vi "LibCam_Open.vi"(7 "webcamnum":i32, 8 "error in (no error)":errorcluster, 10 "height":u32, 11 "width":u32) -> (0 "error out":errorcluster, 3 "return type":i32)   [LabVIEW 2014, in "QwaveSys Raspberry Pi Library.lvlib"]
uses:
  QwaveSys Raspberry Pi Library.lvlib
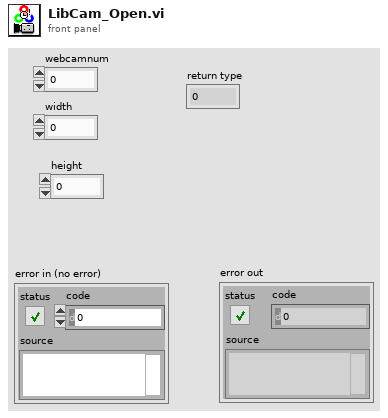
[diagram p1: front panel]
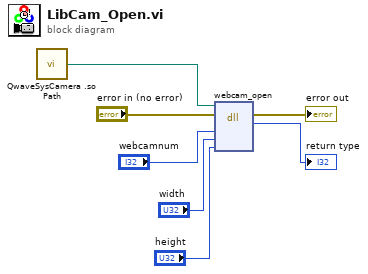
[diagram p0: block diagram]
diagram:
  n1 = call "QwaveSysCamera .so Path.vi"() -> ("QwaveSys .so Path"=w7:path)  [unwired: 5 in]
  n2 = dll-call lib="libcamera.so" fn="webcam_open"(path in=w7, error in="error in (no error)", "camnum"="webcamnum", "w"="width", "h"="height") -> (error out=→"error out":errorcluster, "return type"=→"return type":i32)  [unwired: 4 in, 1 out]
